vi "sub_verifyRows.vi"(11 "puzzle (in)":string[][](array[string])) -> (1 "invalid row":i32, 2 "invalid ?":bool, 3 "solved ?":bool)   [LabVIEW 2018]
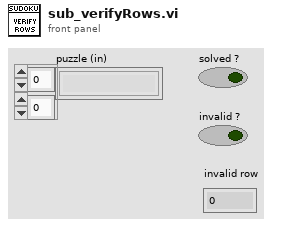
[diagram p1: front panel]
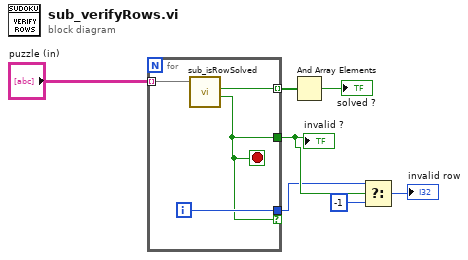
[diagram p0: block diagram]
diagram:
  n1 = for {
    tunnel: "puzzle (in)" -> [w10] mode=indexing
    tunnel: [w11] -> w6 mode=indexing
    tunnel: [w8] -> w4
    tunnel: [w9] -> w3 if=w8
    i -> [w9]
    stop <- w8 stop-if-true
    n2 = call "sub_isRowSolved.vi"("row (in)"=w10) -> ("invalid ?"=w8:bool, "solved ?"=w11:bool)  [unwired: 8 in, 1 out]
  }
  "invalid ?" <- w4
  n3 = And Array Elements(Boolean array=w6) -> (logical AND=→"solved ?":bool)
  n4 = Select(t=w3, s=w4, f=-1) -> (s? t:f=→"invalid row":i32)
